vi "Get Bits (I16).vi"(10 "Bits":u8[](array[numeric]), 11 "Number":i16 format="%.0x") -> (2 "Values":bool[](array[boolean]), 3 "Number Out":i16 format="%.0x")   [LabVIEW 2019, in "Bits.lvlib"]
doc: "Returns the bit value of the bit in the passed in number."
uses:
  Bits.lvlib
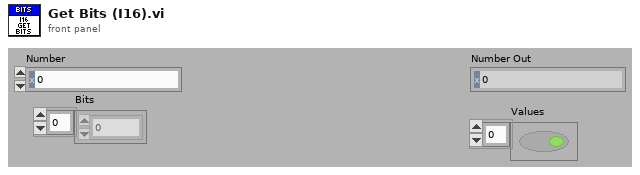
[diagram p1: front panel]
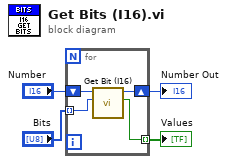
[diagram p0: block diagram]
diagram:
  n1 = for {
    shift-right: [w7] -> w4
    shift-left: "Number" -> [w8]
    tunnel: "Bits" -> [w6] mode=indexing
    tunnel: [w5] -> w1 mode=indexing
    n2 = call "Get Bit (I16).vi"("Bit"=w6, "Number"=w8) -> ("Value"=w5:bool, "Number Out"=w7:i16)  [unwired: 8 in]
  }
  "Values" <- w1
  "Number Out" <- w4
